vi "Workspace.Select.Initialize.vi"(7 "VI reference (current VI)":refnum<vi>, 8 "error in (no error)":errorcluster, 10 "Tree":refnum<vi>, 11 "NIVS.System Definition Root":refnum<k24>) -> (0 "error out":errorcluster, 3 "NIVS.System Definition Root":refnum<k24>)   [LabVIEW 2019, in "Diagnostics Workspace Shared.lvlib"]
uses:
  Diagnostics Workspace Shared.lvlib
  NationalInstruments.VeriStand.SystemStorage
  <vilib>/picture/picture.llb/imagedata.ctl
  Addon/Addon Shared/SubVIs/Constants.vi
  NationalInstruments.VeriStand.SystemDefinitionAPI
  Addon/Addon Shared/Diagnostics Addon Shared.lvlib
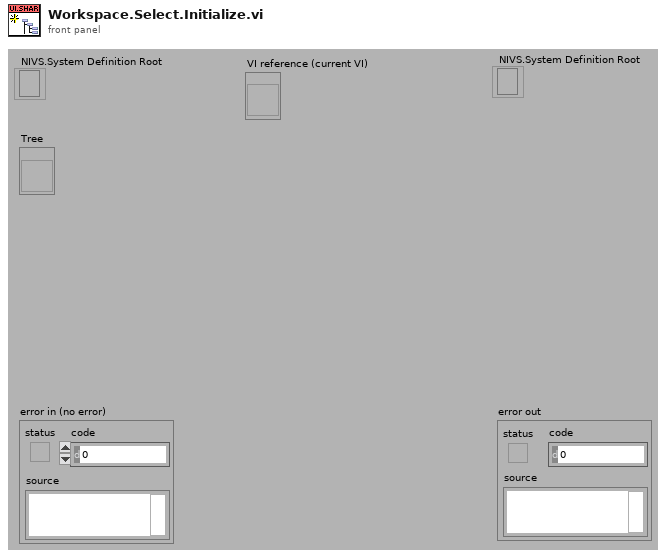
[diagram p1: front panel]
types:
  T1 = typedef "imagedata.ctl" = cluster{"image type":i32, "image depth":i32, "image":u8[], "mask":u8[], "colors":u32[], "Rectangle":cluster{"left":i16, "top":i16, "right":i16, "bottom":i16}}
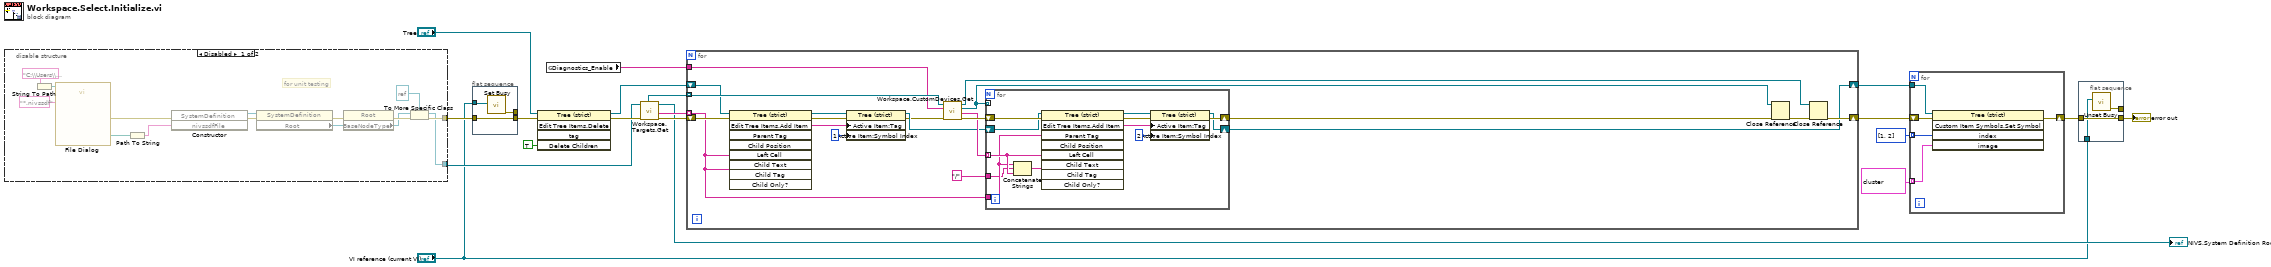
[diagram p0: block diagram]
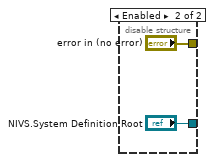
[diagram p2: hidden frame]
diagram:
  n1 = disable-structure shown="Disabled" {
    disable-tunnel: [w21 "NIVS.System Definition Root"] -> w11
    disable-tunnel: [w26 "error in (no error)"] -> w3
    frame Disabled {
      # "for unit testing"
      n2 = String To Path(string="C:\\Users\\Public\\Documents\\National Instruments\\NI VeriStand 2010\\Projects") -> (path=w22:path)
      n3 = call "File Dialog"("start path"=w22, "pattern (all files)"="*.nivssdf") -> ("selected path"=w33:path, "error out"=w20:errorcluster)  [unwired: 10 in, 2 out]
      n4 = Path To String(path=w33) -> (string=w32:string)
      n5 = constructor class="SystemDefinition"(error in=w20, "nivssdfFile"=w32) -> (reference out=w30:refnum<k24>, error out=w31:errorcluster)  [unwired: 2 in, 2 out]
      n6 = property class="SystemDefinition"(reference=w30, error in=w31) -> (error out=w28:errorcluster, "Root"=w29:refnum<k24>)  [unwired: 1 out]
      n7 = property class="Root"(reference=w29, error in=w28) -> (error out=w27:errorcluster, "BaseNodeType"=w25:refnum<k24>)  [unwired: 1 out]
      n8 = To More Specific Class(target class=refnum<k24> refnum, reference=w25, error in=w27) -> (specific class reference=w21:refnum<k24>, error out=w26:errorcluster)
    }
    frame Enabled {
    }
  }
  n9 = flat-sequence {
    tunnel: [w38] -> w17
    tunnel: "VI reference (current VI)" -> [w39]
    tunnel: w3 -> [w38]
    tunnel: [w37] -> _
    frame #0 {
      n10 = call <vilib>:"Set Busy.vi"("VI reference (current VI)"=w39) -> ("error out"=w37:errorcluster)  [unwired: 9 in, 1 out]
    }
  }
  n11 = invoke class="Tree (strict)" method="Edit Tree Items.Delete"(reference="Tree", error in=w17, "Delete Children"=TRUE ("Delete Children?")) -> (reference out=w10:refnum<vi>, error out=w16:errorcluster)  [unwired: 2 in, 3 out]
  n12 = global read "Constants.vi" "Diagnostics_Enable"() -> (w1:string)
  n13 = call "Workspace.Targets.Get.vi"("error in (no error)"=w16, "NIVS.System Definition Root"=w11) -> ("error out"=w15:errorcluster, "Target Names"=w19:string[], "NIVS.System Defintion Root Out"=→"NIVS.System Definition Root":refnum<k24>, "Target Nodes"=w14:refnum<k24>[])  [unwired: 6 in]
  n14 = for {
    tunnel: w14 -> [w58] mode=indexing
    tunnel: w19 -> [w51] mode=indexing
    shift-right: [w53] -> w8
    shift-left: w15 -> [w59]
    tunnel: w1 -> [w49]
    shift-right: [w42] -> w9
    shift-left: w10 -> [w41]
    n15 = invoke class="Tree (strict)" method="Edit Tree Items.Add Item"(reference=w41, error in=w59, "Left Cell"=w51, "Child Tag"=w51) -> (reference out=w47:refnum<vi>, error out=w44:errorcluster, "Edit Tree Items:Add Item"=w45:string)  [unwired: 5 in, 6 out]
    n16 = property class="Tree (strict)"(reference=w47, error in=w44, "Active Item:Tag"=w45, "Active Item:Symbol Index"=1) -> (reference out=w46:refnum<vi>, error out=w43:errorcluster)
    n17 = call "Workspace.CustomDevices.Get.vi"("error in (no error)"=w43, "CD GUID"=w49, "Target Node"=w58) -> ("error out"=w57:errorcluster, "Custom Device Names"=w56:string[], "Custom Device Nodes"=w40:refnum<k24>[], "Target Node Out"=w52:refnum<k24>)  [unwired: 5 in]
    n18 = for {
      tunnel: w56 -> [w70] mode=indexing
      tunnel: w51 -> [w68]
      shift-right: [w61] -> w55
      shift-left: w57 -> [w71]
      tunnel: "/" ("string") -> [w62]
      shift-right: [w60] -> w42
      shift-left: w46 -> [w69]
      tunnel: w40 -> [_] mode=indexing
      n19 = Concatenate Strings(w68, w62, w70) -> (w63:string)
      n20 = invoke class="Tree (strict)" method="Edit Tree Items.Add Item"(reference=w69, error in=w71, "Parent Tag"=w68, "Left Cell"=w70, "Child Tag"=w63) -> (reference out=w66:refnum<vi>, error out=w64:errorcluster, "Edit Tree Items:Add Item"=w65:string)  [unwired: 4 in, 6 out]
      n21 = property class="Tree (strict)"(reference=w66, error in=w64, "Active Item:Tag"=w65, "Active Item:Symbol Index"=2) -> (reference out=w60:refnum<vi>, error out=w61:errorcluster)
    }
    n22 = Close Reference(reference=w40, error in (no error)=w55) -> (error out=w54:errorcluster)
    n23 = Close Reference(reference=w52, error in (no error)=w54) -> (error out=w53:errorcluster)
  }
  n24 = for {
    tunnel: w9 -> [w76]
    shift-right: [w75] -> w6
    shift-left: w8 -> [w73]
    tunnel: i32[] [1, 2] -> [w74] mode=indexing
    tunnel: T1[] [{"image type"=0, "image depth"=32, "image"=array[1024 elements], "mask"=[0, 0, 0, 0, 0, 0, 63, 254, 127, 254, 255, 254, 255, 255, 255, 255, 255, 255, 255, 255, 255, 255, 255, 255, 127, 254, 64, 32, 0, 0, 0, 0], "colors"=[], "Rectangle"={"left"=0, "top"=0, "right"=16, "bottom"=16}}, {"image type"=0, "image depth"=32, "image"=[0, 0, 0, 0, 255, 93, 93, 93, 255, 60, 60, 60, 255, 60, 60, 60, 255, 60, 60, 60, 255, 60, 60, 60, 255, 60, 60, 60, 255, 60, 60, 60, 255, 60, 60, 60, 255, 60, 60, 60, 255, 60, 60, 60, 255, 60, 60, 60, 255, 60, 60, 60, 255, 60, 60, 60, 255, 137, 137, 137, 0, 0, 0, 0, 255, 97, 97, 97, 255, 60, 60, 60, 255, 184, 184, 184, 255, 144, 144, 144, 255, 175, 175, 175, 255, 170, 170, 170, 255, 144, 144, 144, 255, 175, 175, 175, 255, 170, 170, 170, 255, 147, 147, 147, 255, 175, 175, 175, 255, 165, 165, 165, 255, 147, 147, 147, 255, 175, 175, 175, 255, 0, 35, 35, 255, 166, 166, 166, 255, 60, 60, 60, 255, 255, 255, 255, 255, 75, 75, 75, 255, 0, 0, 0, 255, 162, 162, 162, 255, 94, 94, 94, 255, 0, 0, 0, 255, 177, 177, 177, 255, 88, 88, 88, 255, 0, 0, 0, 255, 184, 184, 184, 255, 79, 79, 79, 255, 0, 0, 0, 255, 166, 166, 166, 255, 210, 210, 210, 255, 79, 79, 79, 255, 60, 60, 60, 255, 255, 255, 255, 255, 75, 75, 75, 255, 0, 0, 0, 255, 159, 159, 159, 255, 109, 109, 109, 255, 0, 0, 0, 255, 175, 175, 175, 255, 88, 88, 88, 255, 0, 0, 0, 255, 182, 182, 182, 255, 79, 79, 79, 255, 0, 0, 0, 255, 158, 158, 158, 255, 210, 210, 210, 255, 79, 79, 79, 255, 116, 116, 116, 255, 128, 128, 128, 255, 255, 255, 255, 255, 220, 220, 220, 255, 210, 210, 210, 255, 220, 220, 220, 255, 240, 240, 240, 255, 208, 208, 208, 255, 220, 220, 220, 255, 240, 240, 240, 255, 210, 210, 210, 255, 210, 210, 210, 255, 240, 240, 240, 255, 255, 255, 255, 255, 88, 88, 88, 255, 178, 178, 178, 255, 225, 225, 225, 255, 0, 0, 0, 255, 247, 255, 255, 255, 210, 210, 210, 255, 0, 0, 0, 255, 0, 0, 0, 255, 200, 200, 200, 255, 0, 0, 0, 255, 0, 0, 0, 255, 198, 198, 197, 255, 0, 0, 0, 255, 0, 0, 0, 255, 255, 255, 255, 255, 175, 175, 175, 255, 0, 0, 0, 0, 0, 0, 0, 0, 0, 0, 0, 255, 0, 35, 35, 255, 162, 162, 163, 255, 255, 255, 255, 255, 0, 0, 0, 255, 60, 60, 60, 255, 225, 225, 225, 255, 0, 0, 0, 255, 60, 60, 60, 255, 225, 225, 225, 255, 0, 0, 0, 255, 51, 0, 47, 255, 255, 255, 255, 255, 60, 60, 60, 255, 97, 97, 97, 0, 0, 0, 0, 0, 0, 0, 0, 255, 210, 210, 210, 255, 0, 35, 35, 255, 155, 155, 153, 255, 147, 147, 147, 255, 150, 150, 150, 255, 160, 160, 160, 255, 150, 150, 150, 255, 150, 150, 150, 255, 160, 160, 160, 255, 147, 147, 147, 255, 159, 159, 159, 255, 122, 122, 122, 255, 60, 60, 60, 0, 0, 0, 0, 0, 0, 0, 0, 0, 0, 0, 0, 0, 0, 0, 0, 255, 192, 192, 192, 255, 91, 91, 91, 255, 88, 88, 88, 255, 83, 83, 83, 255, 83, 83, 83, 255, 83, 83, 83, 255, 83, 83, 83, 255, 83, 83, 83, 255, 83, 83, 83, 255, 83, 83, 83, 255, 79, 79, 79, 255, 225, 225, 225, 0, 0, 0, 0, 0, 0, 0, 0], "mask"=[127, 254, 255, 255, 255, 255, 255, 255, 255, 255, 255, 254, 127, 254, 127, 252, 63, 252], "colors"=[], "Rectangle"={"left"=0, "top"=0, "right"=16, "bottom"=9}}] ("Array") -> [w72] mode=indexing
    n25 = invoke on="Invoke Node" class="Tree (strict)" method="Custom Item Symbols.Set Symbol"(reference=w76, error in=w73, "index"=w74, "image"=w72) -> (error out=w75:errorcluster)  [unwired: 1 in, 4 out]
  }
  n26 = flat-sequence {
    tunnel: w6 -> [w79]
    tunnel: [w79] -> w12
    tunnel: [w78] -> _
    tunnel: "VI reference (current VI)" -> [w77]
    frame #0 {
      n27 = call <vilib>:"Unset Busy.vi"("VI reference (current VI)"=w77) -> ("error out"=w78:errorcluster)  [unwired: 10 in]
    }
  }
  "error out" <- w12
